vi "Write Key (Double).vi"(4 "format (fractional)":T1(ring) caption="Format (Dezimalbruch)", 5 "use system decimal point (T)":bool=TRUE caption="Dezimalzeichen des Systems verwenden (T)", 6 "precision (6)":i16=6 caption="Genauigkeit (6)", 7 "section":string caption="Abschnitt", 8 "error in (no error)":errorcluster caption="Fehler (Eingang, kein Fehler)", 9 "value":dbl caption="Wert" format="%.2f", 10 "key":string caption="Schlüssel", 11 "refnum":T2 caption="RefNum") -> (0 "error out":errorcluster caption="Fehler (Ausgang)", 3 "refnum out":T2 caption="RefNum (Ausgang)")   [LabVIEW 2009]
doc: "Schreibt einen Wert, der einem Schlüssel in einem angegebenen Abschnitt in der durch <B>Refnum</B> angegebenen Konfigurationsdatei zugeordnet ist. Mit diesem polymorphen VI können folgende Wertetypen in einen Schlüssel geschrieben werden: boolesche Werte, numerische Werte mit doppelter Genauigkeit, vorzeichenbehaftete Integer-Werte, Pfade, Strings und vorzeichenlose Integer-Werte. Durch den Datentypen, der am Eingang <B>Wert</B> anliegt, wird festgelegt, welche Funktion das polymorphe VI ausführen soll."
uses:
  <vilib>/Utility/config.llb/Config Data RefNum.ctl
  Config Data Modify Functions.ctl
  <vilib>/Utility/config.llb/NI_LVConfig.lvlib
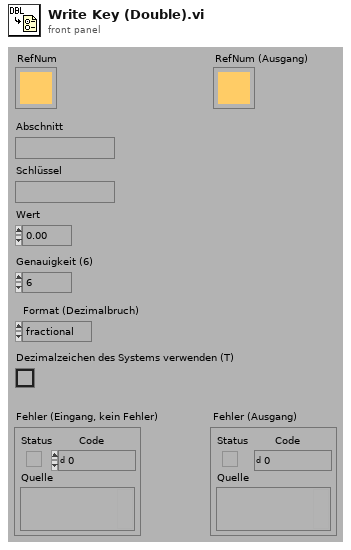
[diagram p1: front panel]
types:
  T1 = enum16{"fractional", "engineering", "exponential"}
  T2 = typedef "NI_LVConfig.lvlib/Config Data RefNum.ctl" = refnum<k1>
  T3 = typedef "Config Data Modify Functions.ctl" = enum16{"set file path", "put data", "add key", "remove section", "remove key"}
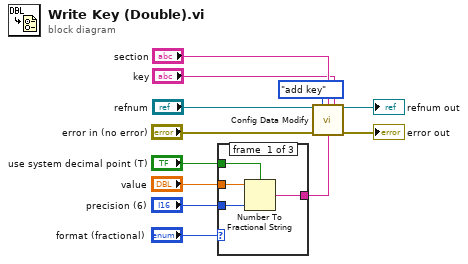
[diagram p0: block diagram]
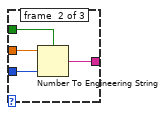
[diagram p2: hidden frame]
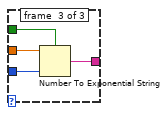
[diagram p3: hidden frame]
diagram:
  n1 = case shown="\"exponential\"" "format (fractional)" {
    tunnel: "value" -> [w16 w20 w24]
    tunnel: "precision (6)" -> [w15 w19 w23]
    tunnel: [w14 w18 w22] -> w3
    tunnel: "use system decimal point (T)" -> [w13 w17 w21]
    frame #0 {
      n2 = Number To Fractional String(use system decimal point (T)=w13, number=w16, precision (6)=w15) -> (F-format string=w14:string)  [unwired: 1 in]
    }
    frame #1 {
      n3 = Number To Engineering String(1:w17, 2:w19, 4:w20) -> (0:w18:string)  [unwired: 1 in]
    }
    frame #2 {
      n4 = Number To Exponential String(number=w24, precision (6)=w23, 1:w21) -> (E-format string=w22:string)  [unwired: 1 in]
    }
  }
  n5 = call "Config Data Modify.vi"("config data"="refnum", "function"=Config_Data_Modify_Functions."add key", "section"="section", "key"="key", "error in (no error)"="error in (no error)", "value"=w3) -> ("config data out"=→"refnum out":T2, "error out"=→"error out":errorcluster)  [unwired: 6 in, 2 out]
